vi "Emballage_BDD_liste valves expediées en txt.vi"(1 "Carton":string[](array[string]), 2 "Liste n° pièces de la cmde":string[](array[string])) -> (0 "liste valves":string="Carton : 1/2\r112105740008030107\r112105740008030106\r112105740008030105\r112105740008030104\r112105740008030103\r112105740008030102\r112105740008030101\r\rCarton : 2/2\r112105740008030110\r112105740008030109\r112105740008030108\r\r")   [LabVIEW 2020]
doc: "Mise en forme txt de la liste des valves emballées par carton pour aller dans la pièce jointe du mail expédition."
panel:
  out "temps Exe [s]":dbl
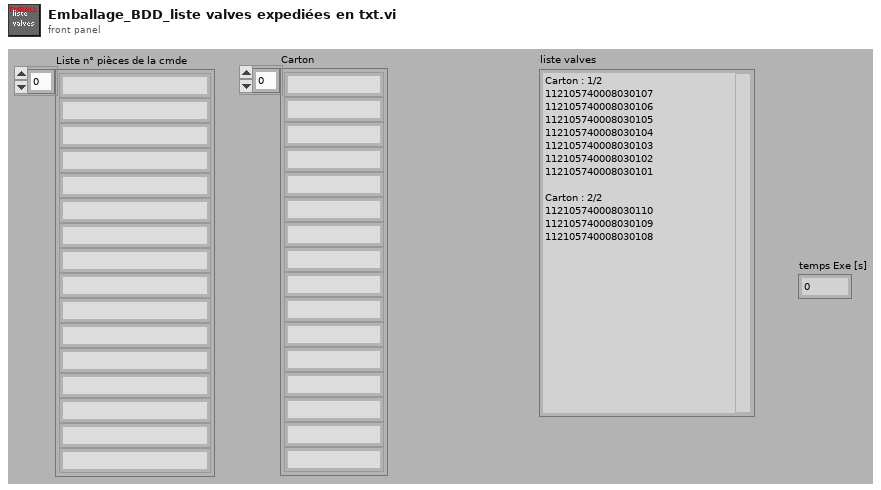
[diagram p1: front panel]
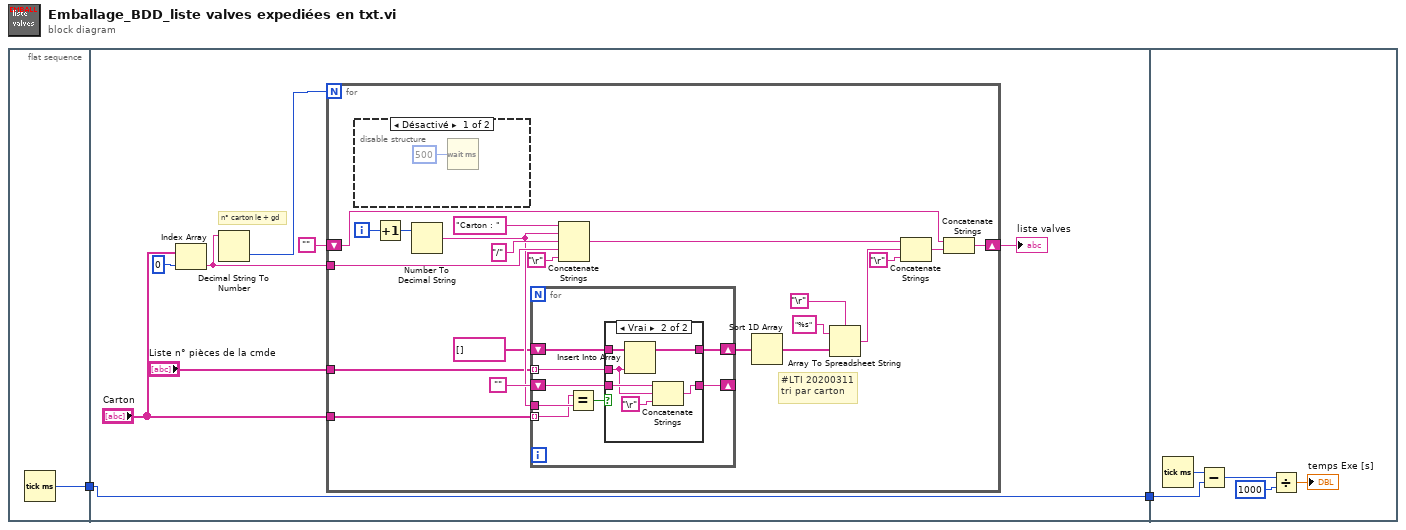
[diagram p0: block diagram]
diagram:
  n1 = flat-sequence {
    tunnel: [w3] -> w1
    tunnel: [w4] -> w2
    tunnel: w1 -> [w4]
    tunnel: w2 -> [w50]
    frame #0 {
      n2 = Tick Count (ms)() -> (millisecond timer value=w3:u32)
    }
    frame #1 {
      # "n° carton le + gd"
      n3 = Index Array(array="Carton", index=0 ("indice")) -> (element=w8:string)
      n4 = Decimal String To Number(string=w8) -> (number=w9:i32)  [unwired: 2 in, 1 out]
      n5 = for {
        N: w9 -> [_]
        tunnel: w8 -> [w26]
        shift-right: [w21] -> w10
        shift-left: "" -> [w20]
        tunnel: "Liste n° pièces de la cmde" -> [w19]
        tunnel: "Carton" -> [w18]
        i -> [w31]
        # "#LTI 20200311\ntri par carton"
        n6 = disable-structure shown="Désactivé" {
          frame Disabled {
            n7 = Wait (ms)(milliseconds to wait=u32 500 ("attente (ms)")) -> ()  [unwired: 1 out]
          }
          frame Enabled {
          }
        }
        n8 = Increment(x=w31) -> (x+1=w32:i32)
        n9 = Number To Decimal String(number=w32) -> (decimal integer string=w25:string)  [unwired: 1 in]
        n10 = for {
          tunnel: w18 -> [w40] mode=indexing
          tunnel: w25 -> [w41]
          shift-right: [w37] -> _
          shift-left: "" -> [w36]
          tunnel: w19 -> [w38] mode=indexing
          shift-right: [w34] -> w16
          shift-left: string[] [] -> [w35]
          n11 = Equal?(x=w40, y=w41) -> (x = y?=w39:bool)
          n12 = case shown="Vrai" w39 {
            tunnel: w38 -> [_ w44]
            tunnel: [w43 w47] -> w37
            tunnel: w36 -> [w43 w49]
            tunnel: w35 -> [w42 w46]
            tunnel: [w42 w45] -> w34
            frame False {
            }
            frame True {
              n13 = Insert Into Array(array=w46, new element=w44) -> (w45:string[])  [unwired: 1 in]
              n14 = Concatenate Strings(w49, w44, "\r") -> (w47:string)
            }
          }
        }
        n15 = Concatenate Strings("Carton : " ("expression régulière"), w25, "/" ("chaîne"), w26, "\r") -> (w23:string)
        n16 = Sort 1D Array(array=w16) -> (sorted array=w15:string[])
        n17 = Array To Spreadsheet String(delimiter (Tab)="\r", array=w15, 3:"%s" ("chaîne de format")) -> (spreadsheet string=w12:string)
        n18 = Concatenate Strings(w23, w12, "\r") -> (w22:string)
        n19 = Concatenate Strings(w20, w22) -> (w21:string)
      }
      "liste valves" <- w10
    }
    frame #2 {
      n20 = Tick Count (ms)() -> (millisecond timer value=w51:u32)
      n21 = Subtract(x=w51, y=w50) -> (x-y=w54:u32)
      n22 = Divide(x=w54, y=u32 1000) -> (x/y=→"temps Exe [s]":dbl)
    }
  }
